vi "Write Data.vi"(8 "error in (no error)":errorcluster, 10 "Data":string, 11 "String Data in":refnum<class "String Data.lvclass">) -> (0 "error out":errorcluster, 3 "String Data out":refnum<class "String Data.lvclass">)   [LabVIEW 2015, in "Base Data Class.lvlib" / "String Data.lvclass"]
uses:
  String Data.lvclass
  String Data.lvclass/String Data.ctl
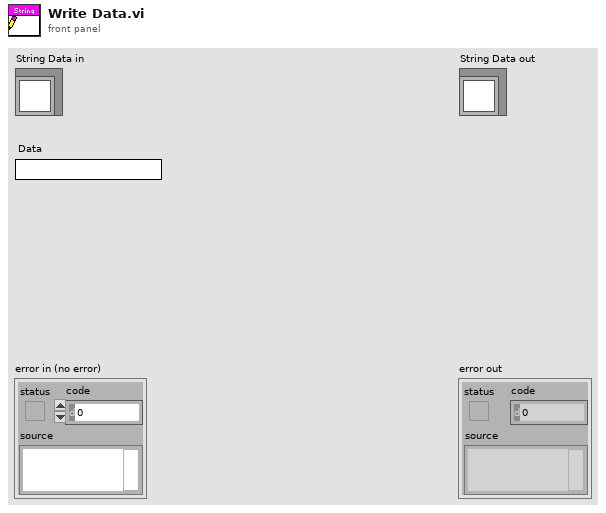
[diagram p1: front panel]
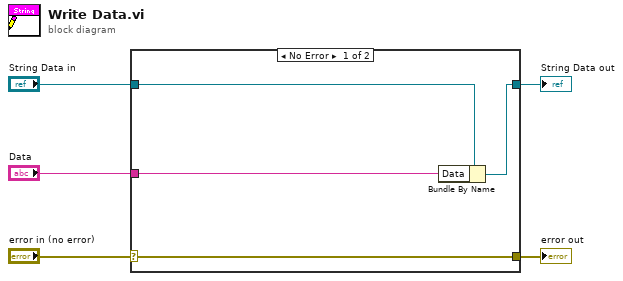
[diagram p0: block diagram]
diagram:
  n1 = case shown="No Error" "error in (no error)" {
    selector: "error in (no error)" -> [w9 w10]
    tunnel: [w9 w10] -> w4
    tunnel: [w7 w11] -> w2
    tunnel: "String Data in" -> [w8 w11]
    tunnel: "Data" -> [w6 _]
    frame No Error {
      n2 = Bundle By Name(cluster=w8, "Data"=w6) -> (w7:refnum<class "String Data.lvclass">)
    }
    frame Error {
    }
  }
  "error out" <- w4
  "String Data out" <- w2
